vi "Mark_NtoS.vi"(1 "Marker(Low->High)":string, 2 "MarkerNumber":u32[](array[numeric])) -> (5 "MarkerString":string[](array[string]))   [LabVIEW 2015, in "ExpData.lvclass"]
uses:
  ExpData.lvclass
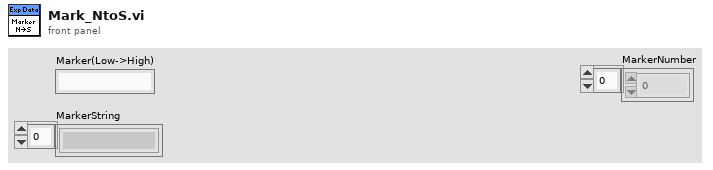
[diagram p1: front panel]
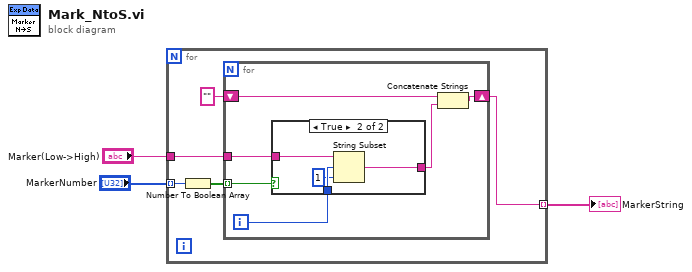
[diagram p0: block diagram]
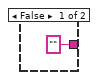
[diagram p2: hidden frame]
diagram:
  n1 = for {
    tunnel: "MarkerNumber" -> [w8] mode=indexing
    tunnel: "Marker(Low->High)" -> [w6]
    tunnel: [w4] -> w1 mode=indexing
    n2 = Number To Boolean Array(number=w8) -> (Boolean array=w7:bool[])
    n3 = for {
      tunnel: w7 -> [w13] mode=indexing
      tunnel: w6 -> [w14]
      shift-right: [w11] -> w4
      shift-left: "" -> [w10]
      i -> [w12]
      n4 = case shown="True" w13 {
        tunnel: w14 -> [_ w19]
        tunnel: w12 -> [_ w18]
        tunnel: ["" ("Marker(Low->High)") w16] -> w9
        frame False {
        }
        frame True {
          n5 = String Subset(string=w19, offset (0)=w18, length (rest)=1 ("length (rest)")) -> (substring=w16:string)
        }
      }
      n6 = Concatenate Strings(w10, w9) -> (w11:string)
    }
  }
  "MarkerString" <- w1
